vi "DAQ Analog In.Async.vi"(10 "Parameters":variant, 11 "Process":refnum<class "Process.lvclass">) -> ()   [LabVIEW 2021, in "DAQ Analog InOut Engine.lvlib"]
uses:
  DAQ Analog InOut Engine.lvlib
  <vilib>/NI/NIVS Inline Async API/_VS Inline Async API/Process/Process.lvclass
  AI Properties.ctl
  System Explorer/Types/Input Channel Parameters.ctl
  <vilib>/NI/NIVS Inline Async API/_VS Inline Async API/Process/Process.lvclass/Process.ctl
  <vilib>/NI/NIVS Inline Async API/_Data Access Engine/Access Type Classes/Write/Write.lvclass/Write.ctl
  <vilib>/NI/NIVS Inline Async API/_Data Access Engine/Data Access Engine/Methods/Write.Data.vi
  <vilib>/DAQmx/read.llb/DAQmx Read (Analog 1D DBL NChan 1Samp).vi
  <vilib>/NI/NIVS Inline Async API/_VS Inline Async API/Process/Data Member Access/Read Data Access.vi
  <vilib>/NI/NIVS Inline Async API/_VS Inline Async API/Error Handling Process/SubVIs/Error.ConvertArray.vi
  <vilib>/NI/NIVS Inline Async API/_Data Access Engine/Access Type Classes/Write/Write.ProcessData.vi
  <vilib>/NI/NIVS Inline Async API/_Data Access Engine/Access Type Classes/Write/Write.Buffer.vi
  <vilib>/NI/NIVS Inline Async API/_Data Access Engine/Access Type Classes/Write/Write.Commit.vi
  <vilib>/NI/NIVS Inline Async API/_Data Access Engine/Data Access Engine/Methods/Write.Lookup.vi
  <vilib>/DAQmx/miscellaneous.llb/DAQmx Fill In Error Info.vi
  <vilib>/NI/NIVS Inline Async API/_Data Access Engine/Data Access Engine/Data Access Engine.lvclass
  System Explorer/DAQ Analog InOut System Explorer.lvlib
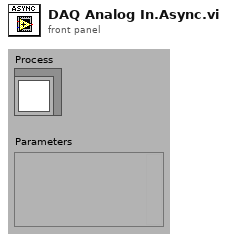
[diagram p1: front panel]
types:
  T1 = typedef "DAQ Analog InOut Engine.lvlib/AI Properties.ctl" = cluster{"AI Channels List":string, "AI Signals properties Array":T2[], "AI Sample Rate":dbl, "AI Signals Array":string[], "PCL Rate [Hz]":dbl, "PCL Decimation":u16}
  T2 = typedef "DAQ Analog InOut System Explorer.lvlib/Input Channel Parameters.ctl" = cluster{"AI MaxV":dbl, "AI MinV":dbl, "Input Configuration":u16}
  T3 = typedef "Data Access Engine.lvlib/Data Access Engine.lvclass/Write.DVR.ctl" = refnum<data-value>
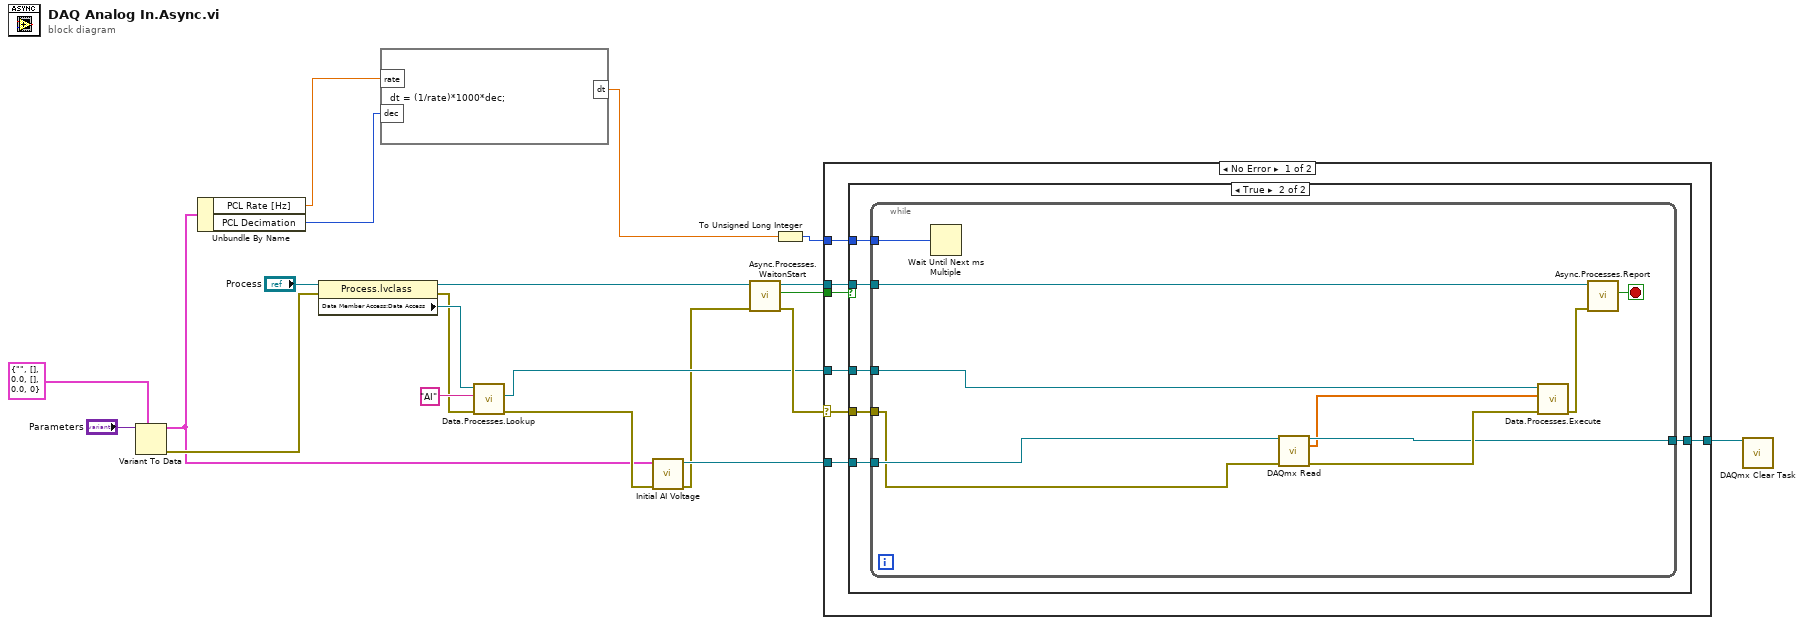
[diagram p0: block diagram]
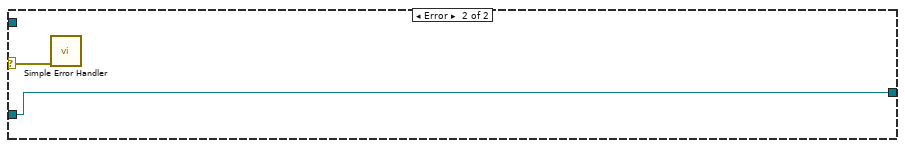
[diagram p3: hidden frame]
diagram:
  n1 = Variant To Data(type=T1 {"AI Channels List"="", "AI Signals properties Array"=[], "AI Sample Rate"=0.0, "AI Signals Array"=[], "PCL Rate [Hz]"=0.0, "PCL Decimation"=0} ("AI Properties"), Variant="Parameters") -> (data=w5:T1, error out=w10:errorcluster)  [unwired: 1 in]
  n2 = Unbundle By Name(w5) -> ("PCL Rate [Hz]"=w4:dbl, "PCL Decimation"=w3:u16)
  n3 = property class="Process.lvclass"(reference="Process", error in=w10) -> (reference out=w15:refnum<class "Process.lvclass">, error out=w13:errorcluster, "Data Member Access:Data Access"=w14:refnum<class "Data Access Engine.lvclass">)
  n4 = formula code="dt = (1/rate)*1000*dec;"("rate"=w4, "dec"=w3) -> ("dt"=w2:dbl)
  n5 = call-poly <vilib>:"Data.Processes.Lookup.vi"("error in (no error)"=w13, "Name"="AI", "Data Access API in"=w14) -> ("error out"=w9:errorcluster, "Ref"=w17:T3)  [unwired: 5 in, 2 out]
  n6 = call "Initial AI Voltage.vi"("error in"=w9, "AI Properties"=w5) -> ("error out"=w6:errorcluster, "DAQ Ref out"=w8:refnum<k21>)  [unwired: 8 in]
  n7 = call <vilib>:"Async.Processes.WaitonStart.vi"("error in (no error)"=w6, "Process"=w15) -> ("error out"=w19:errorcluster, "Execute"=w21:bool, "Process out"=w20:refnum<class "Process.lvclass">)  [unwired: 7 in]
  n8 = To Unsigned Long Integer(number=w2) -> (unsigned 32bit integer=w1:u32)
  n9 = case shown="No Error" w19 {
    selector: w19 -> [w25 w47]
    tunnel: w21 -> [w28 _]
    tunnel: w20 -> [w27 _]
    tunnel: w17 -> [w26 _]
    tunnel: w8 -> [w24 w46]
    tunnel: [w23 w46] -> w7
    tunnel: w1 -> [w22 _]
    frame No Error {
      n10 = case shown="True" w28 {
        tunnel: w25 -> [_ w33]
        tunnel: w27 -> [_ w34]
        tunnel: w26 -> [_ w35]
        tunnel: w24 -> [w29 w32]
        tunnel: [w29 w31] -> w23
        tunnel: w22 -> [_ w30]
        frame False {
        }
        frame True {
          n11 = while {
            tunnel: w33 -> [w38]
            tunnel: w34 -> [w45]
            tunnel: w35 -> [w43]
            tunnel: w32 -> [w41]
            tunnel: [w39] -> w31
            tunnel: w30 -> [w36]
            stop <- w44 stop-if-true
            n12 = Wait Until Next ms Multiple(millisecond multiple=w36) -> ()  [unwired: 1 out]
            n13 = call-poly <vilib>:"DAQmx Read.vi"("task/channels in"=w41, "error in"=w38) -> ("task out"=w39:refnum<k21>, "data"=w37:dbl[], "error out"=w40:errorcluster)  [unwired: 11 in]
            n14 = call-poly <vilib>:"Data.Processes.Execute.vi"("error in (no error)"=w40, "Values"=w37, "Ref"=w43) -> ("error out"=w42:errorcluster)  [unwired: 8 in]
            n15 = call <vilib>:"Async.Processes.Report.vi"("Error"=w42, "Process in"=w45) -> ("Stop"=w44:bool)  [unwired: 8 in, 1 out]
          }
        }
      }
    }
    frame Error {
      n16 = call <vilib>:"Simple Error Handler.vi"("error in (no error)"=w47) -> ()  [unwired: 4 in, 5 out]
    }
  }
  n17 = call <vilib>:"DAQmx Clear Task.vi"("task in"=w7) -> ()  [unwired: 14 in, 1 out]
